vi "Main.vi"() -> ()   [LabVIEW 2020]
uses:
  Code/typeDefs/Parameters.ctl
  Code/typeDefs/MFCIn.ctl
  Code/typeDefs/MFCOut.ctl
  Code/typeDefs/keithleySettings.ctl
  Code/typeDefs/MFCSet.ctl
  <vilib>/Utility/miscctls.llb/LVPointTypeDef.ctl
  <vilib>/DAQmx/read.llb/DAQmx Read (Analog 2D DBL NChan NSamp).vi
  <vilib>/Analysis/baseanly.llb/Mean (DBL).vi
  <vilib>/DAQmx/write.llb/DAQmx Write (Digital 1D Bool NChan 1Samp 1Line).vi
  <vilib>/DAQmx/write.llb/DAQmx Write (Analog DBL 1Chan 1Samp).vi
  <vilib>/DAQmx/create/channels.llb/DAQmx Create Channel (AO-Voltage-Basic).vi
  <vilib>/DAQmx/miscellaneous.llb/DAQmx Fill In Error Info.vi
  <vilib>/DAQmx/create/channels.llb/DAQmx Create Channel (DO-Digital Output).vi
  <vilib>/DAQmx/create/channels.llb/DAQmx Create Channel (AI-Voltage-Basic).vi
  <vilib>/DAQmx/configure/timing.llb/DAQmx Timing (Sample Clock).vi
  <vilib>/Instr/_visa.llb/VISA Configure Serial Port (Instr).vi
  <vilib>/Analysis/NI_AALBase.lvlib
  <resource>/objmgr/daqmx.rc
  Code/DAQ/DAQ.lvclass
  Code/MFC/MFC.lvclass
  Code/SMU/SMU.lvclass
panel:
  out "Residue":dbl
  out "Intercept":dbl
  out "CvsV":T1(graph) caption="Current vs Voltage"
  in  "Timeout Stop":bool
  out "MFC Index":i32
  in  "Names":string[](array[string])=["Resistance (Ohms)", "Ethanol (%)", "RH (%)", "Temp (C)", "MFC A", "MFC B"]
  in  "Stop":bool
  in  "Tab Control":enum32{"Config", "Experiment", "Errors"}(tab)=enum."Experiment"
  in  "AO_LED":tag="6343Sim/ao0"
  in  "DO_Valves":tag="6343Sim/port0/line0:1"
  in  "DAQ channels":tag="6343Sim/ai0:2"
  in  "Keithley 2400 Name":refnum<visa-resource-name>
  in  "MFC Config":T2={"Tare absP"=FALSE, "Tare Flow"=FALSE, "Device ID's"=["A", "B"], "baud rate (9600)"=19200, "VISA COM Port"="COM3"}
  in  "DAQ Config":T3={"RH/T Sensor VSS (V)"=5.048, "K0"=0.9054, "K1"=-2.995, "Offset"=0.0, "Gain"=1.0, "Samples/Channel/s"=1000.0, "Samples to Average"=1000.0} {"Offset" step=0.01 format="%_3f"; "K1" format="%#_13g"; "K0" format="%#_13g"; "RH/T Sensor VSS (V)" format="%.3g"}
  out "Unprocessed Samples in Queue":u32=5
  out "DPS":dbl=100.0 caption="Data Points / Second"
  in  "Keithley Config":T4={"Source Compliance"=0.1, "Min Voltage"=0.0, "Max Voltage"=5.0, "Source Mode"=0, "Number of Points"=50} {"Source Mode" items=["Voltage", "Current"]}
  in  "Keithley Hz":u32=1 min=1 max=100 step=1
  in  "Hours to Run":dbl=1.0 min=0.25 max=10.0 step=0.25 format="%#_5g"
  in  "Aquire data":bool
  out "Start Time":timestamp format="%<%I:%M:%S %p>T"
  in  "MFC Set":T5[](array[typedef])=[{"MFC Set"=[{"String"="A", "MFC set"=1000.0}, {"String"="B", "MFC set"=100.0}], "set 1"=FALSE}, {"MFC Set"=[{"String"="A", "MFC set"=1000.0}, {"String"="B", "MFC set"=100.0}], "set 1"=TRUE}] {"MFC Set"."MFC set" step=10.0 format="%.2f"}
  in  "LED Voltage":dbl(slide) min=0.0 max=10.0 step=0.1 scale=0.0..10.0
  in  "Valves":bool[](array[boolean])=[FALSE, FALSE]
  in  "Plot Data":bool
  out "End Time":timestamp format="%<%I:%M:%S %p>T"
  in  "File Name":string
  in  "Save to File":bool
  out "LED_AO Error":errorcluster
  out "3-Valve_DO Error":errorcluster
  out "DAQ_IO Error":errorcluster
  out "MFC_IO Error":errorcluster
  out "Keithley Error":errorcluster
  in  "Clear I/V":bool
  out "Resistance (ohm)":dbl[](array[numeric])
  in  "Clear DAQ":bool
  out "Array":T6[](array[typedef])=[{"Gas"="", "Setpoint"=0.0, "MassFlow"=0.0, "T ºC"=0.0, "P(PSI)"=0.0, "ID"="-"}, {"Gas"="", "Setpoint"=0.0, "MassFlow"=0.0, "T ºC"=0.0, "P(PSI)"=0.0, "ID"="-"}] {"MassFlow" format="%.2f"; "Setpoint" format="%.2f"}
  out "Waveform Chart":waveform(dbl)[](graph)=[{"t0"=timestamp(3675342615.977705 s since 1904-01-01), "dt"=0.01, "Y"=[0.0007680409200236937]}, {"t0"=timestamp(3675342615.977705 s since 1904-01-01), "dt"=0.01, "Y"=[0.0105205510693704]}, {"t0"=timestamp(3675342615.977705 s since 1904-01-01), "dt"=0.01, "Y"=[89.00820200660893]}, {"t0"=timestamp(3675342615.977705 s since 1904-01-01), "dt"=0.01, "Y"=[117.62674839380017]}, {"t0"=timestamp(3675342615.977705 s since 1904-01-01), "dt"=0.01, "Y"=[0.0]}, {"t0"=timestamp(3675342615.977705 s since 1904-01-01), "dt"=0.01, "Y"=[0.0]}]
  out "T":dbl caption="T  (ºC)" format="%.2g"
  out "RH":dbl caption="RH  (%)" format="%.2g"
  out "Eth":dbl caption="Ethanol (%)" format="%.3g"
  # "Port Config"
  # "Save to File"
  # "1"
  # "2"
  # "1"
  # "2"
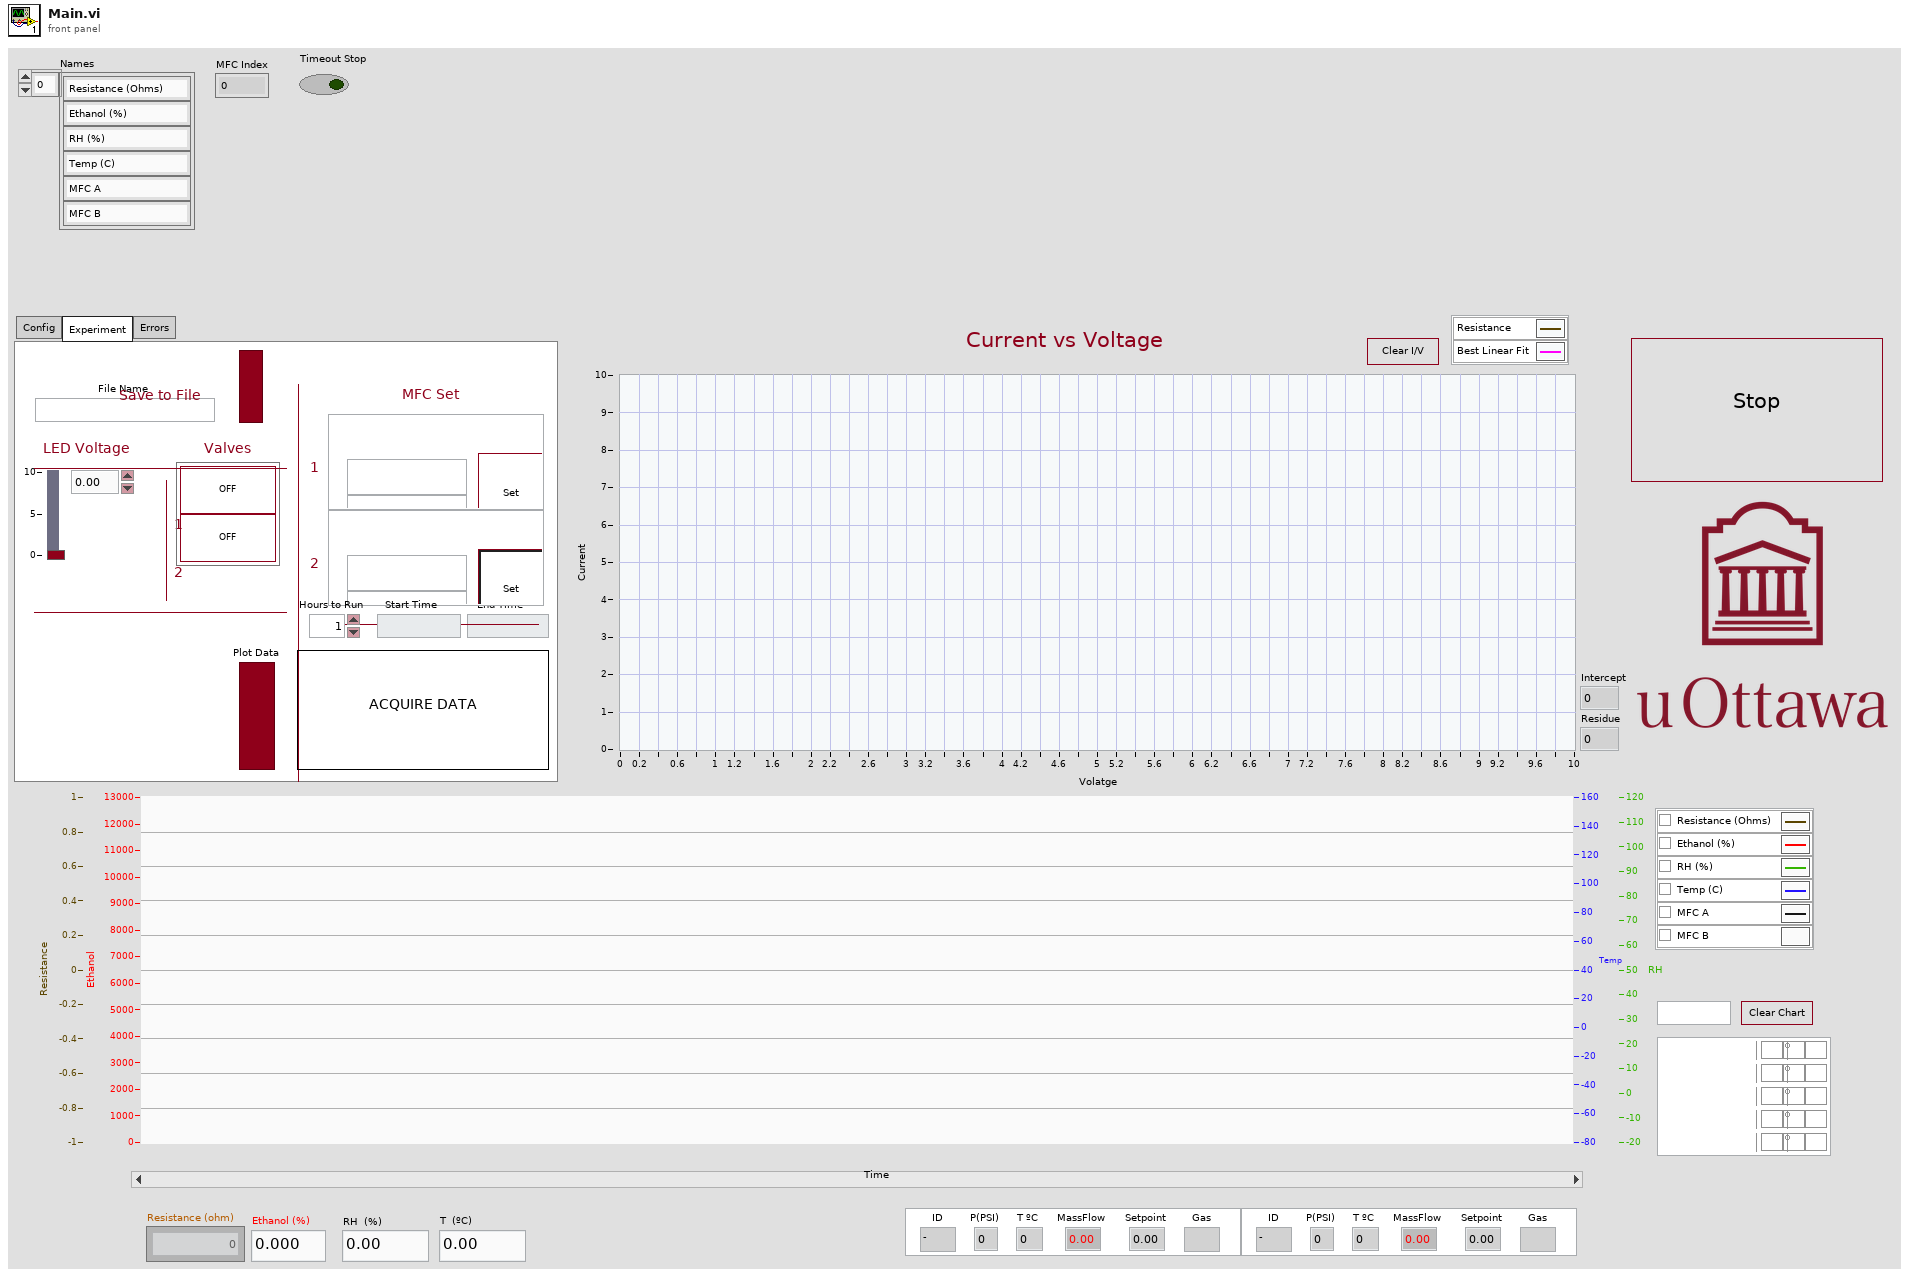
[diagram p1: front panel]
types:
  T1 = cluster{"array":sgl[], "Best Linear Fit":dbl[]}[]
  T2 = typedef "MFCIn.ctl" = cluster{"Tare absP":bool, "Tare Flow":bool, "Device ID's":string[], "baud rate (9600)":u32, "VISA COM Port":refnum<visa-resource-name>}
  T3 = typedef "Parameters.ctl" = cluster{"RH/T Sensor VSS (V)":dbl, "K0":dbl, "K1":dbl, "Offset":dbl, "Gain":dbl, "Samples/Channel/s":dbl, "Samples to Average":dbl}
  T4 = typedef "keithleySettings.ctl" = cluster{"Source Compliance":dbl, "Min Voltage":dbl, "Max Voltage":dbl, "Source Mode":u16, "Number of Points":u32}
  T5 = typedef "MFCSet.ctl" = cluster{"MFC Set":cluster{"String":string, "MFC set":dbl}[], "set 1":bool}
  T6 = typedef "MFCOut.ctl" = cluster{"Gas":string, "Setpoint":dbl, "MassFlow":dbl, "T ºC":dbl, "P(PSI)":dbl, "ID":string}
  T7 = typedef "LVPointTypeDef.ctl" = cluster{"Horizontal":i16, "Vertical":i16}
  T8 = enum8{"Enabled", "Disabled", "Disabled and Grayed Out"}
  T9 = enum32{"invalid app kind", "Development System", "Run Time System", "Student Edition", "Embedded LabVIEW", "Evaluation", "Custom"}
  T10 = cluster{"MFC Set":cluster{"String":bool, "MFC set":bool}[], "set 1":bool}
  T11 = typedef "Graph.ctl" = cluster{"Resistance":dbl, "Ethanol":dbl, "RH":dbl, "Temp":dbl, "MFC A":dbl, "MFC B":dbl}
  T12 = cluster{"ID":string, "P(PSI)":dbl, "T ºC":dbl, "MassFlow":dbl, "Setpoint":dbl, "Gas":string}[]
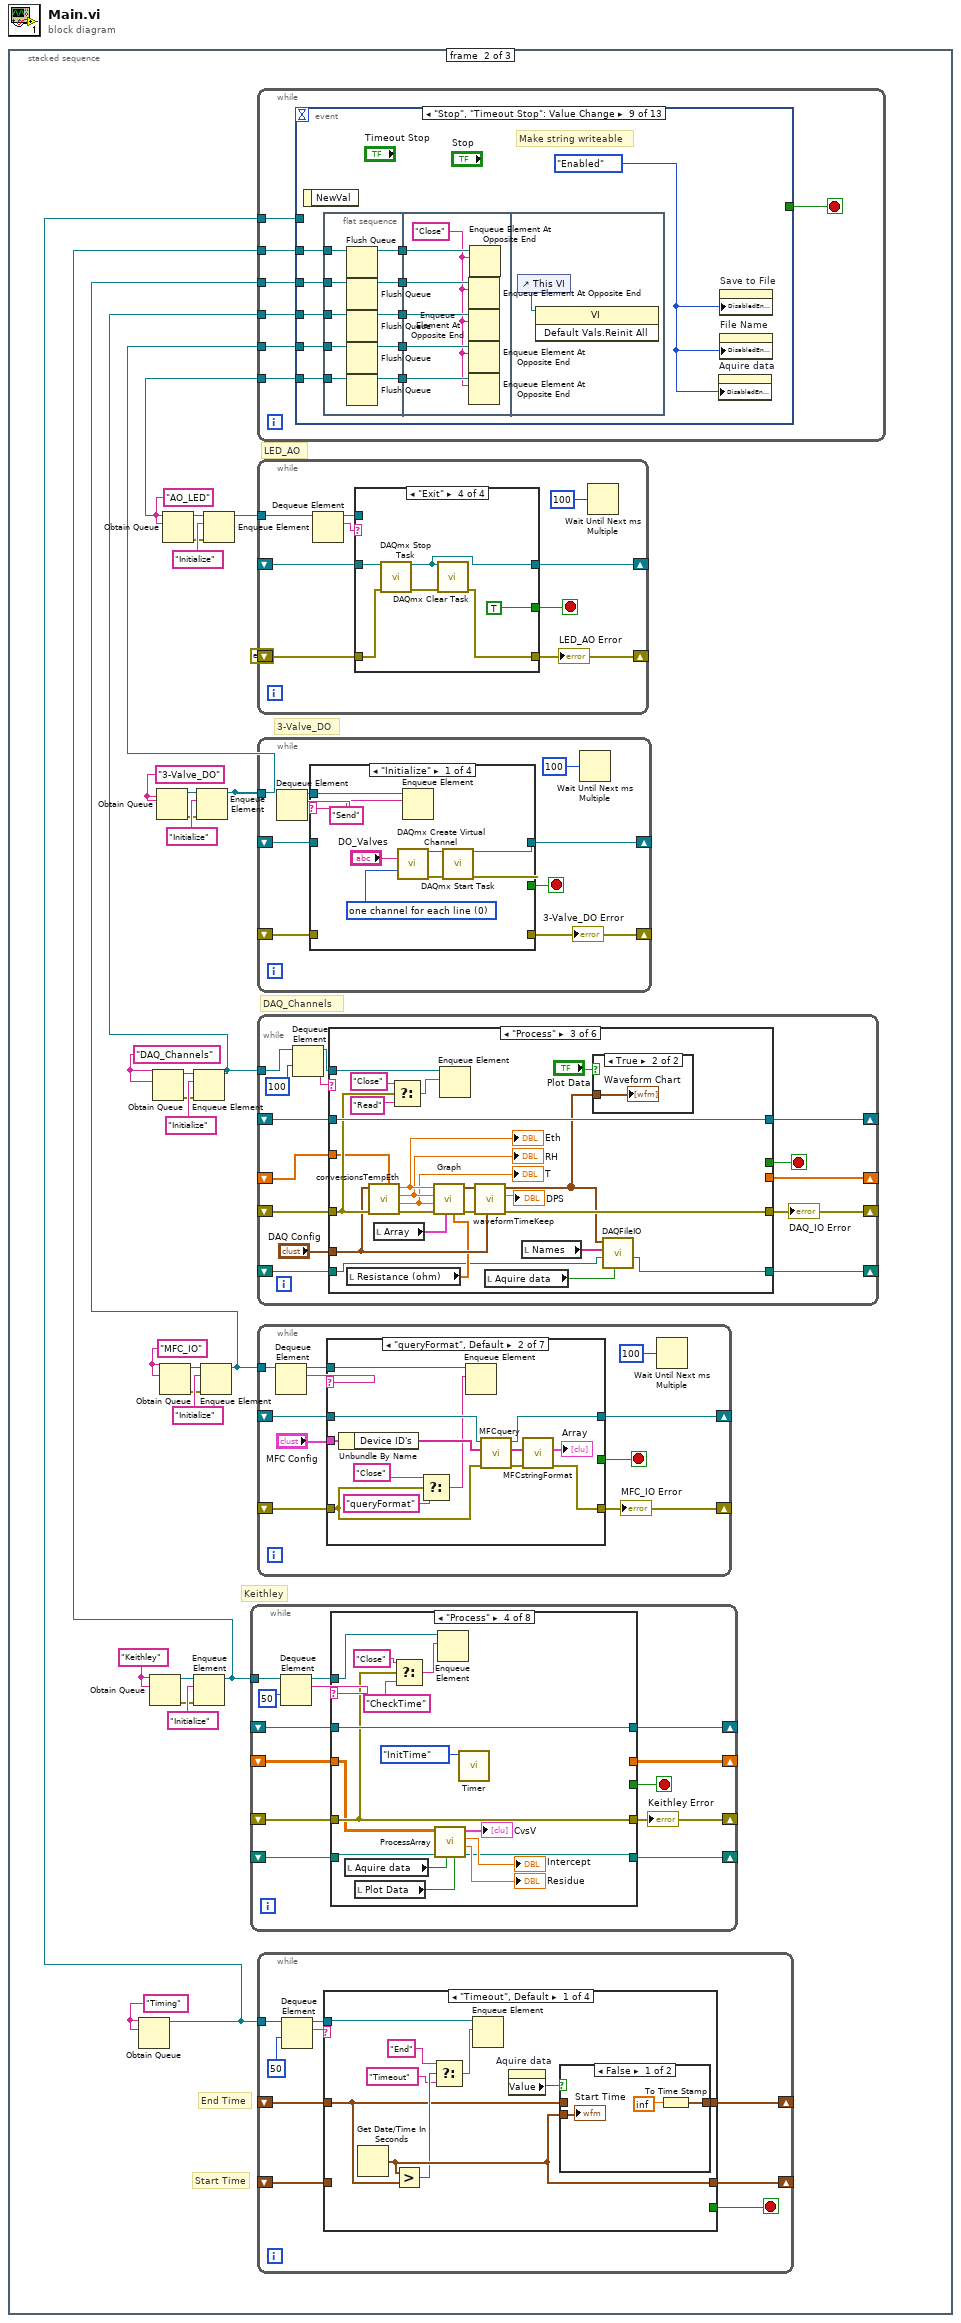
[diagram p0: block diagram]
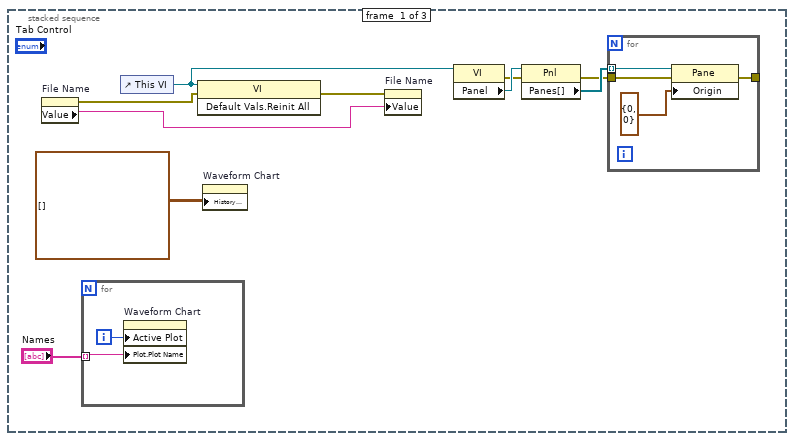
[diagram p2: hidden frame]
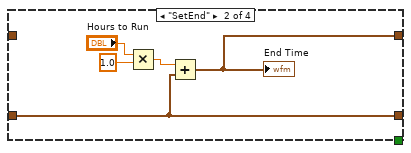
[diagram p4: hidden frame]
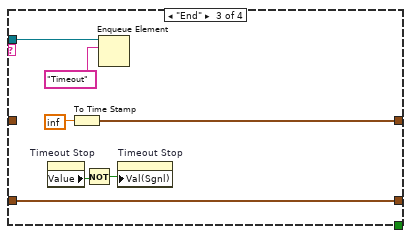
[diagram p5: hidden frame]
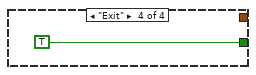
[diagram p6: hidden frame]
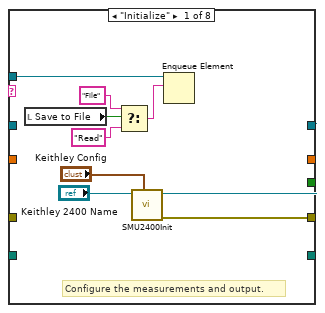
[diagram p7: hidden frame]
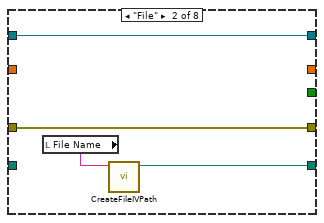
[diagram p8: hidden frame]
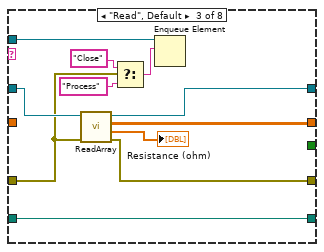
[diagram p9: hidden frame]
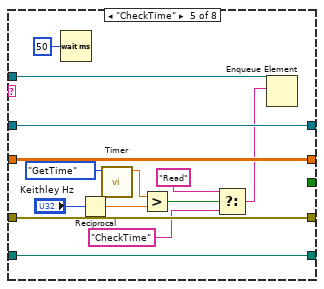
[diagram p10: hidden frame]
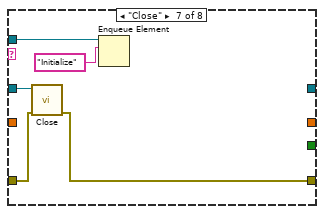
[diagram p12: hidden frame]
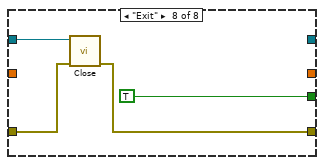
[diagram p13: hidden frame]
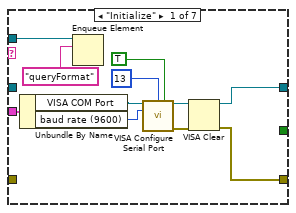
[diagram p14: hidden frame]
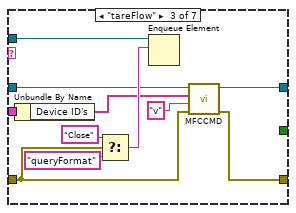
[diagram p15: hidden frame]
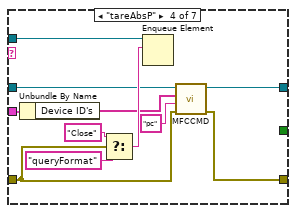
[diagram p16: hidden frame]
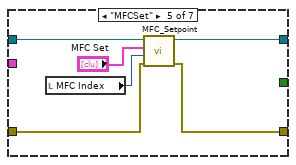
[diagram p17: hidden frame]
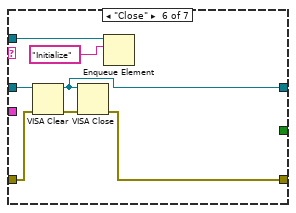
[diagram p18: hidden frame]
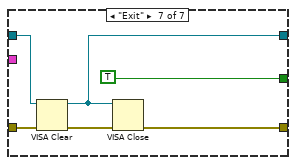
[diagram p19: hidden frame]
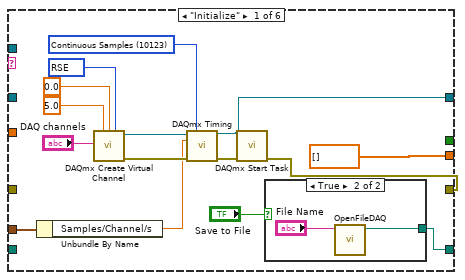
[diagram p20: hidden frame]
diagram:
  n1 = stacked-sequence {
    frame #0 {
      n2 = property on="File Name" class="Str"() -> (error out=w9:errorcluster, "Value"=w8:string)  [unwired: 2 in, 1 out]
      n3 = for {
        tunnel: "Names" -> [w15] mode=indexing
        i -> [w16]
        n4 = property on="Waveform Chart" class="WFChart (strict)"("Active Plot"=w16, "Plot.Plot Name"=w15) -> ()  [unwired: 2 in, 2 out]
      }
      n5 = control-ref of="This VI"() -> (w1:refnum<vi>)
      n6 = invoke class="VI" method="Default Vals.Reinit All"(reference=w1, error in=w9) -> (error out=w7:errorcluster)  [unwired: 1 in, 2 out]
      n7 = property on="Waveform Chart" class="WFChart (strict)"("History Data"=waveform(dbl)[][] []) -> ()  [unwired: 2 in, 2 out]
      n8 = property on="File Name" class="Str"(error in=w7, "Value"=w8) -> ()  [unwired: 1 in, 2 out]
      n9 = property class="VI"(reference=w1) -> (error out=w4:errorcluster, "Panel"=w5:refnum<vi>)  [unwired: 1 in, 1 out]
      n10 = property class="Pnl"(reference=w5, error in=w4) -> (error out=w2:errorcluster, "Panes[]"=w3:refnum<vi>[])  [unwired: 1 out]
      n11 = for {
        tunnel: w3 -> [w14] mode=indexing
        tunnel: w2 -> [w13]
        tunnel: [w11] -> _
        n12 = property class="Pane"(reference=w14, error in=w13, "Origin"=T7 {"Horizontal"=0, "Vertical"=0}) -> (error out=w11:errorcluster)  [unwired: 1 out]
      }
    }
    frame #1 {
      w18 = "Timing" ("name (unnamed)")
      w27 = "Keithley" ("name (unnamed)")
      w31 = "MFC_IO" ("name (unnamed)")
      w34 = "DAQ_Channels" ("name (unnamed)")
      w32 = "3-Valve_DO" ("name (unnamed)")
      w42 = "AO_LED" ("name (unnamed)")
      # "Start Time"
      # "End Time"
      # "Keithley"
      # "DAQ_Channels"
      # "3-Valve_DO"
      # "LED_AO"
      n13 = Obtain Queue(name (unnamed)=w18, element data type=w18) -> (queue out=w17:refnum<queue>)  [unwired: 3 in, 2 out]
      n14 = Obtain Queue(name (unnamed)=w27, element data type=w27) -> (queue out=w21:refnum<queue>, error out=w19:errorcluster)  [unwired: 3 in, 1 out]
      n15 = Obtain Queue(name (unnamed)=w34, element data type=w34) -> (queue out=w26:refnum<queue>, error out=w33:errorcluster)  [unwired: 3 in, 1 out]
      n16 = Obtain Queue(name (unnamed)=w32, element data type=w32) -> (queue out=w36:refnum<queue>, error out=w37:errorcluster)  [unwired: 3 in, 1 out]
      n17 = Obtain Queue(name (unnamed)=w31, element data type=w31) -> (queue out=w29:refnum<queue>, error out=w30:errorcluster)  [unwired: 3 in, 1 out]
      n18 = Obtain Queue(name (unnamed)=w42, element data type=w42) -> (queue out=w40:refnum<queue>, error out=w41:errorcluster)  [unwired: 3 in, 1 out]
      n19 = Enqueue Element(queue=w26, element="Initialize", error in (no error)=w33) -> (queue out=w25:refnum<queue>)  [unwired: 1 in, 2 out]
      n20 = Enqueue Element(queue=w21, element="Initialize", error in (no error)=w19) -> (queue out=w20:refnum<queue>)  [unwired: 1 in, 2 out]
      n21 = Enqueue Element(queue=w36, element="Initialize", error in (no error)=w37) -> (queue out=w22:refnum<queue>)  [unwired: 1 in, 2 out]
      n22 = Enqueue Element(queue=w29, element="Initialize", error in (no error)=w30) -> (queue out=w28:refnum<queue>)  [unwired: 1 in, 2 out]
      n23 = Enqueue Element(queue=w40, element="Initialize", error in (no error)=w41) -> (queue out=w23:refnum<queue>)  [unwired: 1 in, 2 out]
      n24 = while {
        shift-right: [w86] -> _
        shift-left: _ -> [w90]
        shift-right: [w89] -> _
        shift-left: _ -> [w88]
        tunnel: w20 -> [w87]
        shift-right: [w84] -> _
        shift-left: _ -> [w83]
        shift-right: [w82] -> _
        shift-left: _ -> [w81]
        stop <- w85 stop-if-true
        n25 = Dequeue Element(queue=w87, timeout in ms (-1)=50) -> (queue out=w92:refnum<queue>, element=w91:string)  [unwired: 1 in, 2 out]
        n26 = case shown="\"Process\"" w91 {
          tunnel: w92 -> [w101 _ w116 w129 w132 _ w152 _]
          tunnel: [_ _ _ _ _ _ _ TRUE] -> w85
          tunnel: [w94 w105 w107 w126 w145 w148 w151 w155] -> w86
          tunnel: w90 -> [_ w105 w106 w126 w145 w148 w150 w154]
          tunnel: [w93 w103 w109 w127 w138 w147 _ _] -> w89
          tunnel: w88 -> [_ w103 w110 w127 w138 w147 w149 w156]
          tunnel: [_ _ w111 _ w137 _ _ _] -> w84
          tunnel: w83 -> [_ _ _ w123 w137 _ _ _]
          tunnel: [_ w102 w112 w117 w139 w146 _ _] -> w82
          tunnel: w81 -> [_ _ w112 w124 w139 w146 _ _]
          frame "Initialize" {
            # "Configure the measurements and output."
            n27 = local read "Save to File"() -> (w98:bool)
            n28 = Select(t="File", s=w98, f="Read" ("element")) -> (s? t:f=w97:string)
            n29 = call "SMU2400Init.vi"("Keithley Config"="Keithley Config", "Keithley 2400 Name"="Keithley 2400 Name") -> ("error out"=w94:errorcluster, "VISA resource name out"=w93:refnum<visa-resource-name>)  [unwired: 8 in]
            n30 = Enqueue Element(queue=w101, element=w97) -> ()  [unwired: 2 in, 3 out]
          }
          frame "File" {
            n31 = local read "File Name"() -> (w104:string)
            n32 = call "CreateFileIVPath.vi"("File Name"=w104) -> ("appended path"=w102:path)  [unwired: 9 in, 1 out]
          }
          frame "Read", Default {
            n33 = call "ReadArray.vi"("error in (no error)"=w106, "VISA resource name"=w110) -> ("error out"=w107:errorcluster, "Resistance (ohm)"=→"Resistance (ohm)":dbl[], "appended array"=w111:sgl[][], "VISA resource name out"=w109:refnum<visa-resource-name>)  [unwired: 6 in]
            n34 = Select(t="Close" ("element"), s=w106, f="Process" ("element")) -> (s? t:f=w114:string)
            n35 = Enqueue Element(queue=w116, element=w114) -> ()  [unwired: 2 in, 3 out]
          }
          frame "Process" {
            n36 = local read "Aquire data"() -> (w121:bool)
            n37 = local read "Plot Data"() -> (w120:bool)
            n38 = Select(t="Close" ("element"), s=w126, f="CheckTime" ("element")) -> (s? t:f=w128:string)
            n39 = call "ProcessArray.vi"("Plot Data"=w120, "Aquire Data"=w121, "File Path In"=w124, "array in"=w123) -> ("file path out"=w117:path, "residue"=→"Residue":dbl, "intercept"=→"Intercept":dbl, "Array out"=→"CvsV":T1)  [unwired: 4 in]
            n40 = Enqueue Element(queue=w129, element=w128) -> ()  [unwired: 2 in, 3 out]
            n41 = call "Timer.vi"("State"=enum16{"GetTime", "InitTime"}."InitTime") -> ()  [unwired: 10 in, 1 out]
          }
          frame "CheckTime" {
            n42 = Wait (ms)(milliseconds to wait=u32 50) -> ()  [unwired: 1 out]
            n43 = Reciprocal(x="Keithley Hz") -> (1/x=w141:dbl)
            n44 = call "Timer.vi"("State"=enum16{"GetTime", "InitTime"}."GetTime") -> ("Timer (s)"=w142:dbl)  [unwired: 10 in]
            n45 = Greater?(x=w142, y=w141) -> (0:w136:bool)
            n46 = Select(t="Read", s=w136, f="CheckTime") -> (s? t:f=w133:string)
            n47 = Enqueue Element(queue=w132, element=w133) -> ()  [unwired: 2 in, 3 out]
          }
          frame "Clear" {
          }
          frame "Close" {
            n48 = call "Close.vi"("error in (no error)"=w150, "VISA resource name"=w149) -> ("error out"=w151:errorcluster)  [unwired: 8 in, 1 out]
            n49 = Enqueue Element(queue=w152, element="Initialize") -> ()  [unwired: 2 in, 3 out]
          }
          frame "Exit" {
            n50 = call "Close.vi"("error in (no error)"=w154, "VISA resource name"=w156) -> ("error out"=w155:errorcluster)  [unwired: 8 in, 1 out]
          }
        }
        "Keithley Error" <- w86
      }
      n51 = while {
        tunnel: w23 -> [w408]
        tunnel: w22 -> [w407]
        tunnel: w25 -> [w406]
        tunnel: w28 -> [w405]
        tunnel: w20 -> [w404]
        tunnel: w17 -> [w403]
        stop <- w409 stop-if-true
        n52 = event shown="[8] \"Stop\", \"Timeout Stop\": Value Change" {
          selector: _ -> [_ _ _ _ _ _ _ _ _ _ _ _ _]
          dyn-events: _ -> [_ _ _ _ _ _ _ _ _ _ _ _ _]
          timeout: _ -> [_ _ _ _ _ _ _ _ _ _ _ _ _]
          tunnel: [_ _ w416 _ _ _ _ _ _ _ _ _ _] -> w409
          tunnel: w408 -> [_ _ w417 _ _ _ _ _ w457 _ _ _ _]
          tunnel: w407 -> [_ _ w418 _ _ _ _ _ w458 _ _ _ _]
          tunnel: w406 -> [_ _ w419 w433 w437 _ _ _ w459 _ w492 w503 w517]
          tunnel: w405 -> [_ _ w420 _ _ _ w448 w449 w460 w480 _ _ _]
          tunnel: w404 -> [_ _ w421 _ w435 w446 _ _ w461 _ w491 w502 w518]
          tunnel: w403 -> [_ w410 w415 _ _ _ _ _ _ _ _ _ _]
          event Timeout {
            n53 = event-data() -> ()  [unwired: 1 in, 1 out]
          }
          event "Aquire data": Value Change {
            n54 = event-data() -> ("NewVal"=w411:bool)  [unwired: 1 in]
            n55 = case shown="True" w411 {
              tunnel: w410 -> [_ w413]
              frame False {
              }
              frame True {
                w412 = T8."Disabled and Grayed Out" ("Disabled")
                n56 = Enqueue Element(queue=w413, element="SetEnd") -> ()  [unwired: 2 in, 3 out]
                n57 = property on="File Name" class="Str"("DisabledEnum"=w412) -> ()  [unwired: 2 in, 2 out]
                n58 = property on="Aquire data" class="Bool (strict)"("DisabledEnum"=w412) -> ()  [unwired: 2 in, 2 out]
                n59 = property on="Save to File" class="Bool (strict)"("DisabledEnum"=w412) -> ()  [unwired: 2 in, 2 out]
              }
            }
          }
          event Panel Close? {
            n60 = event-data() -> ()  [unwired: 1 in, 1 out]
            n61 = Two Button Dialog(message="Are you sure you would like to close?", 2:"Yes" ("T button name (\"OK\")")) -> (T button?=w416:bool)  [unwired: 1 in]
            n62 = case shown="True" w416 {
              tunnel: w421 -> [_ w431]
              tunnel: w420 -> [_ w430]
              tunnel: w419 -> [_ w429]
              tunnel: w418 -> [_ w428]
              tunnel: w417 -> [_ w427]
              tunnel: w415 -> [_ w426]
              frame False {
              }
              frame True {
                w425 = "Exit" ("element")
                n63 = Enqueue Element At Opposite End(queue=w430, element=w425) -> ()  [unwired: 2 in, 3 out]
                n64 = Enqueue Element At Opposite End(queue=w429, element=w425) -> ()  [unwired: 2 in, 3 out]
                n65 = Enqueue Element At Opposite End(queue=w428, element=w425) -> ()  [unwired: 2 in, 3 out]
                n66 = Enqueue Element At Opposite End(queue=w427, element=w425) -> ()  [unwired: 2 in, 3 out]
                n67 = Enqueue Element At Opposite End(queue=w426, element=w425) -> ()  [unwired: 2 in, 3 out]
                n68 = Enqueue Element At Opposite End(queue=w431, element=w425) -> ()  [unwired: 2 in, 3 out]
              }
            }
            n69 = event-data("Discard?"=TRUE) -> ()  [unwired: 1 in, 1 out]
          }
          event "Clear DAQ": Value Change {
            n70 = event-data() -> ()  [unwired: 1 in, 1 out]
            n71 = Enqueue Element(queue=w433, element="Clear") -> ()  [unwired: 2 in, 3 out]
          }
          event Value Change {
            n72 = event-data() -> ()  [unwired: 1 in, 1 out]
            n73 = flat-sequence {
              tunnel: w437 -> [w441]
              tunnel: [w440] -> w436
              tunnel: w435 -> [w439]
              tunnel: [w438] -> w434
              tunnel: w436 -> [w444]
              tunnel: w434 -> [w443]
              frame #0 {
                n74 = Flush Queue(queue=w441) -> (queue out=w440:refnum<queue>)  [unwired: 1 in, 2 out]
                n75 = Flush Queue(queue=w439) -> (queue out=w438:refnum<queue>)  [unwired: 1 in, 2 out]
              }
              frame #1 {
                w442 = "Close" ("element")
                n76 = Enqueue Element(queue=w444, element=w442) -> ()  [unwired: 2 in, 3 out]
                n77 = Enqueue Element(queue=w443, element=w442) -> ()  [unwired: 2 in, 3 out]
              }
            }
          }
          event "Clear I/V": Value Change {
            n78 = event-data() -> ()  [unwired: 1 in, 1 out]
            n79 = Enqueue Element(queue=w446, element="Clear") -> ()  [unwired: 2 in, 3 out]
          }
          event Value Change {
            n80 = event-data() -> ()  [unwired: 1 in, 6 out]
            n81 = Enqueue Element(queue=w448, element="tareFlow") -> ()  [unwired: 2 in, 3 out]
          }
          event Value Change {
            n82 = event-data() -> ()  [unwired: 1 in, 1 out]
            n83 = Enqueue Element(queue=w449, element="tareAbsP") -> ()  [unwired: 2 in, 3 out]
          }
          event "Stop", "Timeout Stop": Value Change {
            w451 = T8."Enabled" ("Disabled")
            # "Make string writeable"
            n84 = event-data() -> ()  [unwired: 1 in, 1 out]
            n85 = flat-sequence {
              tunnel: w457 -> [w463]
              tunnel: w458 -> [w465]
              tunnel: w459 -> [w467]
              tunnel: w460 -> [w469]
              tunnel: w461 -> [w471]
              tunnel: [w470] -> w456
              tunnel: [w468] -> w455
              tunnel: [w466] -> w454
              tunnel: [w464] -> w453
              tunnel: [w462] -> w452
              tunnel: w456 -> [w477]
              tunnel: w455 -> [w473]
              tunnel: w454 -> [w474]
              tunnel: w453 -> [w475]
              tunnel: w452 -> [w476]
              frame #0 {
                n86 = Flush Queue(queue=w471) -> (queue out=w470:refnum<queue>)  [unwired: 1 in, 2 out]
                n87 = Flush Queue(queue=w469) -> (queue out=w468:refnum<queue>)  [unwired: 1 in, 2 out]
                n88 = Flush Queue(queue=w467) -> (queue out=w466:refnum<queue>)  [unwired: 1 in, 2 out]
                n89 = Flush Queue(queue=w465) -> (queue out=w464:refnum<queue>)  [unwired: 1 in, 2 out]
                n90 = Flush Queue(queue=w463) -> (queue out=w462:refnum<queue>)  [unwired: 1 in, 2 out]
              }
              frame #1 {
                w472 = "Close" ("element")
                n91 = Enqueue Element At Opposite End(queue=w473, element=w472) -> ()  [unwired: 2 in, 3 out]
                n92 = Enqueue Element At Opposite End(queue=w474, element=w472) -> ()  [unwired: 2 in, 3 out]
                n93 = Enqueue Element At Opposite End(queue=w475, element=w472) -> ()  [unwired: 2 in, 3 out]
                n94 = Enqueue Element At Opposite End(queue=w476, element=w472) -> ()  [unwired: 2 in, 3 out]
                n95 = Enqueue Element At Opposite End(queue=w477, element=w472) -> ()  [unwired: 2 in, 3 out]
              }
              frame #2 {
                n96 = control-ref of="This VI"() -> (w478:refnum<vi>)
                n97 = invoke class="VI" method="Default Vals.Reinit All"(reference=w478) -> ()  [unwired: 2 in, 3 out]
              }
            }
            n98 = property on="Aquire data" class="Bool (strict)"("DisabledEnum"=w451) -> ()  [unwired: 2 in, 2 out]
            n99 = property on="Save to File" class="Bool (strict)"("DisabledEnum"=w451) -> ()  [unwired: 2 in, 2 out]
            n100 = property on="File Name" class="Str"("DisabledEnum"=w451) -> ()  [unwired: 2 in, 2 out]
          }
          event "MFC Set": Value Change {
            n101 = event-data() -> ("OldVal"=w481:T5[], "NewVal"=w479:T5[])  [unwired: 1 in]
            n102 = for {
              tunnel: w481 -> [w487] mode=indexing
              tunnel: w480 -> [w483]
              tunnel: w479 -> [w482] mode=indexing
              i -> [w485]
              stop <- w484 stop-if-true
              n103 = Not Equal?(x=w487, y=w482) -> (x != y?=w486:T10)
              n104 = Unbundle(w486) -> ("set 1"=w484:bool)  [unwired: 1 out]
              n105 = case shown="True" w484 {
                tunnel: w483 -> [_ w488]
                frame False {
                }
                frame True {
                  n106 = Enqueue Element(queue=w488, element="MFCSet") -> ()  [unwired: 2 in, 3 out]
                }
              }
              "MFC Index" <- w485
            }
          }
          event "File Name": Value Change {
            n107 = event-data() -> ()  [unwired: 1 in, 1 out]
            n108 = flat-sequence {
              tunnel: w492 -> [w497]
              tunnel: [w496] -> w493
              tunnel: w491 -> [w495]
              tunnel: [w494] -> w490
              tunnel: w493 -> [w500]
              tunnel: w490 -> [w499]
              frame #0 {
                n109 = Flush Queue(queue=w497) -> (queue out=w496:refnum<queue>)  [unwired: 1 in, 2 out]
                n110 = Flush Queue(queue=w495) -> (queue out=w494:refnum<queue>)  [unwired: 1 in, 2 out]
              }
              frame #1 {
                w498 = "Close" ("element")
                n111 = Enqueue Element(queue=w500, element=w498) -> ()  [unwired: 2 in, 3 out]
                n112 = Enqueue Element(queue=w499, element=w498) -> ()  [unwired: 2 in, 3 out]
              }
            }
          }
          event "Save to File": Value Change {
            n113 = event-data() -> ("NewVal"=w506:bool)  [unwired: 1 in]
            n114 = flat-sequence {
              tunnel: w503 -> [w510]
              tunnel: [w509] -> w504
              tunnel: w502 -> [w508]
              tunnel: [w507] -> w501
              tunnel: w504 -> [w513]
              tunnel: w501 -> [w512]
              frame #0 {
                n115 = Flush Queue(queue=w510) -> (queue out=w509:refnum<queue>)  [unwired: 1 in, 2 out]
                n116 = Flush Queue(queue=w508) -> (queue out=w507:refnum<queue>)  [unwired: 1 in, 2 out]
              }
              frame #1 {
                w511 = "Close" ("element")
                n117 = Enqueue Element(queue=w512, element=w511) -> ()  [unwired: 2 in, 3 out]
                n118 = Enqueue Element(queue=w513, element=w511) -> ()  [unwired: 2 in, 3 out]
              }
            }
            n119 = case shown="False" w506 {
              tunnel: [T8."Enabled" ("Disabled") T8."Disabled and Grayed Out" ("Disabled")] -> w505
              frame False {
              }
              frame True {
              }
            }
            n120 = property on="File Name" class="Str"("DisabledEnum"=w505) -> ()  [unwired: 2 in, 2 out]
          }
          event Value Change {
            n121 = event-data() -> ()  [unwired: 1 in, 1 out]
            n122 = flat-sequence {
              tunnel: w518 -> [w523]
              tunnel: [w522] -> w519
              tunnel: w517 -> [w521]
              tunnel: [w520] -> w516
              tunnel: w519 -> [w526]
              tunnel: w516 -> [w525]
              frame #0 {
                n123 = Flush Queue(queue=w523) -> (queue out=w522:refnum<queue>)  [unwired: 1 in, 2 out]
                n124 = Flush Queue(queue=w521) -> (queue out=w520:refnum<queue>)  [unwired: 1 in, 2 out]
              }
              frame #1 {
                w524 = "Close" ("element")
                n125 = Enqueue Element(queue=w525, element=w524) -> ()  [unwired: 2 in, 3 out]
                n126 = Enqueue Element(queue=w526, element=w524) -> ()  [unwired: 2 in, 3 out]
              }
            }
          }
        }
      }
      n127 = while {
        shift-right: [w367] -> _
        shift-left: errorcluster {"status"=FALSE, "code"=0, "source"=""} ("error out") -> [w370]
        shift-right: [w369] -> _
        shift-left: _ -> [w368]
        tunnel: w23 -> [w366]
        stop <- w371 stop-if-true
        n128 = Dequeue Element(queue=w366) -> (queue out=w373:refnum<queue>, element=w372:string)  [unwired: 2 in, 2 out]
        n129 = case shown="\"Exit\"" w372 {
          tunnel: w373 -> [w380 w389 w395 _]
          tunnel: [_ _ _ TRUE] -> w371
          tunnel: [w377 w386 w392 w400] -> w367
          tunnel: w370 -> [_ w385 w390 w398]
          tunnel: [w378 w387 w393 w397] -> w369
          tunnel: w368 -> [_ w388 w394 w401]
          frame "Initialize" {
            n130 = Enqueue Element(queue=w380, element="Send") -> ()  [unwired: 2 in, 3 out]
            n131 = call-poly <vilib>:"DAQmx Create Virtual Channel.vi"("physical channels"="AO_LED") -> ("task out"=w376:refnum<k21>, "error out"=w375:errorcluster)  [unwired: 13 in]
            n132 = call <vilib>:"DAQmx Start Task.vi"("task/channels in"=w376, "error in"=w375) -> ("task out"=w378:refnum<k21>, "error out"=w377:errorcluster)  [unwired: 12 in]
          }
          frame "Send", Default {
            n133 = Select(t="Close" ("element"), s=w385, f="Send" ("element")) -> (s? t:f=w382:string)
            n134 = call-poly <vilib>:"DAQmx Write.vi"("task/channels in"=w388, "data"="LED Voltage", "error in"=w385) -> ("task out"=w387:refnum<k21>, "error out"=w386:errorcluster)  [unwired: 10 in, 1 out]
            n135 = Enqueue Element(queue=w389, element=w382) -> ()  [unwired: 2 in, 3 out]
          }
          frame "Close" {
            n136 = call <vilib>:"DAQmx Stop Task.vi"("task/channels in"=w394, "error in"=w390) -> ("task out"=w393:refnum<k21>, "error out"=w391:errorcluster)  [unwired: 12 in]
            n137 = call <vilib>:"DAQmx Clear Task.vi"("task in"=w393, "error in"=w391) -> ("error out"=w392:errorcluster)  [unwired: 13 in]
            n138 = Enqueue Element(queue=w395, element="Initialize") -> ()  [unwired: 2 in, 3 out]
          }
          frame "Exit" {
            n139 = call <vilib>:"DAQmx Stop Task.vi"("task/channels in"=w401, "error in"=w398) -> ("task out"=w397:refnum<k21>, "error out"=w399:errorcluster)  [unwired: 12 in]
            n140 = call <vilib>:"DAQmx Clear Task.vi"("task in"=w397, "error in"=w399) -> ("error out"=w400:errorcluster)  [unwired: 13 in]
          }
        }
        "LED_AO Error" <- w367
        n141 = Wait Until Next ms Multiple(millisecond multiple=u32 100) -> ()  [unwired: 1 out]
      }
      n142 = while {
        shift-right: [w327] -> _
        shift-left: _ -> [w330]
        shift-right: [w329] -> _
        shift-left: _ -> [w328]
        tunnel: w22 -> [w326]
        stop <- w332 stop-if-true
        n143 = Dequeue Element(queue=w326) -> (queue out=w334:refnum<queue>, element=w333:string)  [unwired: 2 in, 2 out]
        n144 = case shown="\"Initialize\"" w333 {
          tunnel: w334 -> [w342 w351 w357 _]
          tunnel: [_ _ _ TRUE] -> w332
          tunnel: [w339 w348 w354 w361] -> w327
          tunnel: w330 -> [_ w347 w352 w359]
          tunnel: [w340 w349 w355 w362] -> w329
          tunnel: w328 -> [_ w350 w356 w363]
          frame "Initialize" {
            w336 = 0 items=["one channel for each line", "one channel for all lines"] ("line grouping")
            n145 = call-poly <vilib>:"DAQmx Create Virtual Channel.vi"("lines"="DO_Valves", "line grouping"=w336) -> ("task out"=w338:refnum<k21>, "error out"=w337:errorcluster)  [unwired: 12 in]
            n146 = Enqueue Element(queue=w342, element="Send") -> ()  [unwired: 2 in, 3 out]
            n147 = call <vilib>:"DAQmx Start Task.vi"("task/channels in"=w338, "error in"=w337) -> ("task out"=w340:refnum<k21>, "error out"=w339:errorcluster)  [unwired: 12 in]
          }
          frame "Send", Default {
            n148 = Select(t="Close" ("element"), s=w347, f="Send" ("element")) -> (s? t:f=w344:string)
            n149 = Enqueue Element(queue=w351, element=w344) -> ()  [unwired: 2 in, 3 out]
            n150 = call-poly <vilib>:"DAQmx Write.vi"("task/channels in"=w350, "data"="Valves", "error in"=w347) -> ("task out"=w349:refnum<k21>, "error out"=w348:errorcluster)  [unwired: 10 in, 1 out]
          }
          frame "Close" {
            n151 = call <vilib>:"DAQmx Stop Task.vi"("task/channels in"=w356, "error in"=w352) -> ("task out"=w355:refnum<k21>, "error out"=w353:errorcluster)  [unwired: 12 in]
            n152 = call <vilib>:"DAQmx Clear Task.vi"("task in"=w355, "error in"=w353) -> ("error out"=w354:errorcluster)  [unwired: 13 in]
            n153 = Enqueue Element(queue=w357, element="Initialize") -> ()  [unwired: 2 in, 3 out]
          }
          frame "Exit" {
            n154 = call <vilib>:"DAQmx Stop Task.vi"("task/channels in"=w363, "error in"=w359) -> ("task out"=w362:refnum<k21>, "error out"=w360:errorcluster)  [unwired: 12 in]
            n155 = call <vilib>:"DAQmx Clear Task.vi"("task in"=w362, "error in"=w360) -> ("error out"=w361:errorcluster)  [unwired: 13 in]
          }
        }
        "3-Valve_DO Error" <- w327
        n156 = Wait Until Next ms Multiple(millisecond multiple=u32 100) -> ()  [unwired: 1 out]
      }
      n157 = while {
        shift-right: [w241] -> _
        shift-left: _ -> [w244]
        shift-right: [w243] -> _
        shift-left: _ -> [w242]
        shift-right: [w240] -> _
        shift-left: _ -> [w238]
        tunnel: w25 -> [w239]
        shift-right: [w234] -> _
        shift-left: _ -> [w233]
        stop <- w236 stop-if-true
        n158 = Dequeue Element(queue=w239, timeout in ms (-1)=100) -> (queue out=w246:refnum<queue>, element=w245:string)  [unwired: 1 in, 2 out]
        n159 = case shown="\"Process\"" w245 {
          tunnel: w246 -> [_ w273 w304 _ w315 _]
          tunnel: [_ _ _ _ _ TRUE] -> w236
          tunnel: [w248 w267 w294 w311 w313 w323] -> w241
          tunnel: w244 -> [_ w270 w301 w309 w314 w320]
          tunnel: [w254 w276 w302 w312 _ _] -> w243
          tunnel: w242 -> [_ w278 w302 w312 w316 w324]
          tunnel: [dbl[] [] w269 _ dbl[] [] _ _] -> w240
          tunnel: w238 -> [_ _ w292 _ _ _]
          tunnel: "DAQ Config" -> [w252 w265 w289 _ _ _]
          tunnel: [w247 w264 w285 w307 _ _] -> w234
          tunnel: w233 -> [_ w264 w282 w307 _ _]
          frame "Initialize" {
            w257 = 10123 items=["Finite Samples"=10178, "Continuous Samples"=10123, "Hardware Timed Single Point"=12522] ("sample mode")
            w250 = 10083 items=["default"=-1, "RSE"=10083, "NRSE"=10078, "Differential"=10106, "Pseudodifferential"=12529] ("input terminal configuration")
            n160 = Unbundle By Name(w252) -> ("Samples/Channel/s"=w251:dbl)
            n161 = call-poly <vilib>:"DAQmx Create Virtual Channel.vi"("maximum value"=5.0, "minimum value"=0.0, "input terminal configuration"=w250, "physical channels"="DAQ channels") -> ("task out"=w258:refnum<k21>, "error out"=w259:errorcluster)  [unwired: 10 in]
            n162 = call-poly <vilib>:"DAQmx Timing.vi"("task/channels in"=w258, "sample mode"=w257, "rate"=w251, "error in"=w259) -> ("task out"=w254:refnum<k21>, "error out"=w260:errorcluster)  [unwired: 10 in]
            n163 = call <vilib>:"DAQmx Start Task.vi"("task/channels in"=w254, "error in"=w260) -> ("error out"=w248:errorcluster)  [unwired: 12 in, 1 out]
            n164 = case shown="True" "Save to File" {
              tunnel: [_ w262] -> w247
              frame False {
              }
              frame True {
                n165 = call "OpenFileDAQ.vi"("DAQ File Name"="File Name") -> ("appended path"=w262:path)  [unwired: 8 in, 1 out]
              }
            }
          }
          frame "Read", Default {
            n166 = Unbundle By Name(w265) -> ("Samples to Average"=w275:dbl)
            n167 = property class="DAQmx Read"(reference=w278, error in=w270) -> (reference out=w277:refnum<k21>, error out=w274:errorcluster, "AvailSampPerChan"=→"Unprocessed Samples in Queue":u32)
            n168 = Select(t="Close" ("element"), s=w270, f="Process" ("element")) -> (s? t:f=w279:string)
            n169 = Enqueue Element(queue=w273, element=w279) -> ()  [unwired: 2 in, 3 out]
            n170 = call-poly <vilib>:"DAQmx Read.vi"("task/channels in"=w277, "number of samples per channel"=w275, "error in"=w274) -> ("task out"=w276:refnum<k21>, "data"=w268:dbl[][], "error out"=w267:errorcluster)  [unwired: 10 in]
            n171 = for {
              tunnel: w268 -> [w280] mode=indexing
              tunnel: [w281] -> w269 mode=indexing
              n172 = call-poly <vilib>:"Mean.vi"("X"=w280) -> ("mean"=w281:dbl)  [unwired: 1 out]
            }
          }
          frame "Process" {
            n173 = local read "Resistance (ohm)"() -> (w287:dbl[])
            n174 = call "conversionsTempEth.vi"("Array"=w292, "error in (no error)"=w301, "Parameters"=w289) -> ("error out"=w299:errorcluster, "T"=w296:dbl, "RH"=w297:dbl, "Ethanol"=w298:dbl)  [unwired: 5 in]
            "Eth" <- w298
            "RH" <- w297
            "T" <- w296
            n175 = local read "Array"() -> (w300:T6[])
            n176 = Select(t="Close" ("element"), s=w301, f="Read") -> (s? t:f=w303:string)
            n177 = call "Graph.vi"("Resistance"=w287, "Array in"=w300, "error in (no error)"=w299, "T  (ºC)"=w296, "RH  (%)"=w297, "Ethanol (%)"=w298) -> ("error out"=w295:errorcluster, "Cluster"=w293:T11)  [unwired: 4 in]
            n178 = Enqueue Element(queue=w304, element=w303) -> ()  [unwired: 2 in, 3 out]
            n179 = call "waveformTimeKeep.vi"("DAQ Settings"=w289, "error in (no error)"=w295, "input cluster"=w293) -> ("error out"=w294:errorcluster, "Samples/second"=→"DPS":dbl, "appended array"=w283:waveform(dbl)[])  [unwired: 6 in]
            n180 = local read "Aquire data"() -> (w286:bool)
            n181 = local read "Names"() -> (w284:string[])
            n182 = case shown="True" "Plot Data" {
              tunnel: w283 -> [_ w306]
              frame False {
              }
              frame True {
                "Waveform Chart" <- w306
              }
            }
            n183 = call "DAQFileIO.vi"("Aquire Data"=w286, "File Path In"=w282, "Names"=w284, "data"=w283) -> ("file path out"=w285:path)  [unwired: 6 in, 1 out]
          }
          frame "Clear" {
            n184 = property on="Waveform Chart" class="WFChart (strict)"(error in=w309, "History Data"=waveform(dbl)[][] []) -> (error out=w311:errorcluster)  [unwired: 1 in, 1 out]
          }
          frame "Close" {
            n185 = call <vilib>:"DAQmx Stop Task.vi"("task/channels in"=w316, "error in"=w314) -> ("task out"=w317:refnum<k21>, "error out"=w318:errorcluster)  [unwired: 12 in]
            n186 = Enqueue Element(queue=w315, element="Initialize") -> ()  [unwired: 2 in, 3 out]
            n187 = call <vilib>:"DAQmx Clear Task.vi"("task in"=w317, "error in"=w318) -> ("error out"=w313:errorcluster)  [unwired: 13 in]
          }
          frame "Exit" {
            n188 = call <vilib>:"DAQmx Stop Task.vi"("task/channels in"=w324, "error in"=w320) -> ("task out"=w321:refnum<k21>, "error out"=w322:errorcluster)  [unwired: 12 in]
            n189 = call <vilib>:"DAQmx Clear Task.vi"("task in"=w321, "error in"=w322) -> ("error out"=w323:errorcluster)  [unwired: 13 in]
          }
        }
        "DAQ_IO Error" <- w241
      }
      n190 = while {
        shift-right: [w161] -> _
        shift-left: _ -> [w164]
        shift-right: [w163] -> _
        shift-left: _ -> [w162]
        tunnel: w28 -> [w160]
        stop <- w165 stop-if-true
        n191 = Dequeue Element(queue=w160) -> (queue out=w167:refnum<queue>, element=w166:string)  [unwired: 2 in, 2 out]
        n192 = case shown="\"queryFormat\", Default" w166 {
          tunnel: w167 -> [w177 w186 w195 w205 _ w225 _]
          tunnel: [_ _ _ _ _ _ TRUE] -> w165
          tunnel: [w170 w179 w200 w207 w218 w221 w231] -> w161
          tunnel: w164 -> [_ w189 w193 w208 w219 w223 w229]
          tunnel: [w169 w184 w196 w203 w216 w220 w227] -> w163
          tunnel: w162 -> [_ w188 w197 w204 w217 w224 w228]
          tunnel: "MFC Config" -> [w175 w183 w199 w206 _ _ _]
          frame "Initialize" {
            n193 = Unbundle By Name(w175) -> ("VISA COM Port"=w174:refnum<visa-resource-name>, "baud rate (9600)"=w173:u32)
            n194 = Enqueue Element(queue=w177, element="queryFormat") -> ()  [unwired: 2 in, 3 out]
            n195 = call-poly "VISA Configure Serial Port"("VISA resource name"=w174, "termination char\n(0xA = '\\n' = LF)"=u8 13 ("termination char\n(0xA = '\\n' = LF)"), "Enable Termination\nChar (T)"=TRUE ("Enable Termination\nChar (T)"), "baud rate (9600)"=w173) -> ("VISA resource name out"=w176:refnum<visa-resource-name>, "error out"=w168:errorcluster)  [unwired: 10 in]
            n196 = VISA Clear(VISA resource name=w176, error in (no error)=w168) -> (VISA resource name out=w169:refnum<visa-resource-name>, error out=w170:errorcluster)
          }
          frame "queryFormat", Default {
            n197 = Unbundle By Name(w183) -> ("Device ID's"=w187:string[])
            n198 = Select(t="Close" ("element"), s=w189, f="queryFormat" ("element")) -> (s? t:f=w185:string)
            n199 = Enqueue Element(queue=w186, element=w185) -> ()  [unwired: 2 in, 3 out]
            n200 = call "MFCquery.vi"("error in (no error)"=w189, "Device ID's"=w187, "VISA Refnum in"=w188) -> ("error out"=w180:errorcluster, "Array"=w182:string[], "VISA Refnum out"=w184:refnum<visa-resource-name>)  [unwired: 6 in]
            n201 = call "MFCstringFormat.vi"("error in (no error)"=w180, "Array"=w182) -> ("error out"=w179:errorcluster, "Array out"=→"Array":T12)  [unwired: 7 in]
          }
          frame "tareFlow" {
            n202 = Unbundle By Name(w199) -> ("Device ID's"=w198:string[])
            n203 = Select(t="Close" ("element"), s=w193, f="queryFormat" ("element")) -> (s? t:f=w202:string)
            n204 = Enqueue Element(queue=w195, element=w202) -> ()  [unwired: 2 in, 3 out]
            n205 = call "MFCCMD.vi"("error in (no error)"=w193, "cmd"="v", "Device ID's"=w198, "VISA Refnum in"=w197) -> ("error out"=w200:errorcluster, "VISA Refnum out"=w196:refnum<visa-resource-name>)  [unwired: 6 in]
          }
          frame "tareAbsP" {
            n206 = Unbundle By Name(w206) -> ("Device ID's"=w212:string[])
            n207 = Select(t="Close" ("element"), s=w208, f="queryFormat" ("element")) -> (s? t:f=w213:string)
            n208 = Enqueue Element(queue=w205, element=w213) -> ()  [unwired: 2 in, 3 out]
            n209 = call "MFCCMD.vi"("error in (no error)"=w208, "cmd"="pc", "Device ID's"=w212, "VISA Refnum in"=w204) -> ("error out"=w207:errorcluster, "VISA Refnum out"=w203:refnum<visa-resource-name>)  [unwired: 6 in]
          }
          frame "MFCSet" {
            n210 = local read "MFC Index"() -> (w215:i32)
            n211 = call "MFC_Setpoint.vi"("error in"=w219, "index"=w215, "MFC Set"="MFC Set", "VISA Refnum in"=w217) -> ("error out"=w218:errorcluster, "VISA Refnum out"=w216:refnum<visa-resource-name>)  [unwired: 6 in]
          }
          frame "Close" {
            n212 = VISA Clear(VISA resource name=w224, error in (no error)=w223) -> (VISA resource name out=w220:refnum<visa-resource-name>, error out=w222:errorcluster)
            n213 = VISA Close(VISA resource name=w220, error in (no error)=w222) -> (error out=w221:errorcluster)
            n214 = Enqueue Element(queue=w225, element="Initialize") -> ()  [unwired: 2 in, 3 out]
          }
          frame "Exit" {
            n215 = VISA Clear(VISA resource name=w228, error in (no error)=w229) -> (VISA resource name out=w227:refnum<visa-resource-name>, error out=w230:errorcluster)
            n216 = VISA Close(VISA resource name=w227, error in (no error)=w230) -> (error out=w231:errorcluster)
          }
        }
        "MFC_IO Error" <- w161
        n217 = Wait Until Next ms Multiple(millisecond multiple=u32 100) -> ()  [unwired: 1 out]
      }
      n218 = while {
        tunnel: w17 -> [w53]
        shift-right: [w49] -> _
        shift-left: _ -> [w46]
        shift-right: [w48] -> _
        shift-left: _ -> [w47]
        stop <- w45 stop-if-true
        n219 = Dequeue Element(queue=w53, timeout in ms (-1)=50) -> (queue out=w51:refnum<queue>, element=w52:string)  [unwired: 1 in, 2 out]
        n220 = case shown="\"Timeout\", Default" w52 {
          tunnel: w51 -> [w55 _ w75 _]
          tunnel: [w60 w67 w78 _] -> w49
          tunnel: [w61 w68 w76 _] -> w48
          tunnel: w47 -> [w54 _ _ _]
          tunnel: w46 -> [_ w67 w78 _]
          tunnel: [_ _ _ TRUE] -> w45
          frame "Timeout", Default {
            n221 = Get Date/Time In Seconds() -> (seconds since 1Jan1904=w60:timestamp)
            n222 = Greater?(x=w60, y=w54) -> (0:w59:bool)
            n223 = Select(t="End" ("element"), s=w59, f="Timeout" ("element")) -> (s? t:f=w58:string)
            n224 = Enqueue Element(queue=w55, element=w58) -> ()  [unwired: 2 in, 3 out]
            n225 = property on="Aquire data" class="Bool (strict)"() -> ("Value"=w62:bool)  [unwired: 2 in, 2 out]
            n226 = case shown="False" w62 {
              tunnel: [w63 w66] -> w61
              tunnel: w60 -> [w65 _]
              tunnel: w54 -> [_ w66]
              frame False {
                n227 = To Time Stamp(1:inf) -> (0:w63:timestamp)
                "Start Time" <- w65
              }
              frame True {
              }
            }
          }
          frame "SetEnd" {
            n228 = Multiply(x="Hours to Run", y=1.0) -> (x*y=w69:dbl)
            n229 = Add(x=w69, y=w67) -> (x+y=w68:timestamp)
            "End Time" <- w68
          }
          frame "End" {
            n230 = property on="Timeout Stop" class="Bool (strict)"() -> ("Value"=w73:bool)  [unwired: 2 in, 2 out]
            n231 = To Time Stamp(1:inf) -> (0:w76:timestamp)
            n232 = Not(x=w73) -> (.not. x?=w72:bool)
            n233 = Enqueue Element(queue=w75, element="Timeout") -> ()  [unwired: 2 in, 3 out]
            n234 = property on="Timeout Stop" class="Bool (strict)"("Val(Sgnl)"=w72) -> ()  [unwired: 2 in, 2 out]
          }
          frame "Exit" {
          }
        }
      }
    }
    frame #2 {
      # "In development environment, do not close the panel"
      n235 = property class="App"() -> ("App.Kind"=w528:T9)  [unwired: 2 in, 2 out]
      n236 = Equal?(x=w528, y=T9."Run Time System" ("Application:Kind")) -> (x = y?=w529:bool)
      n237 = case shown="True" w529 {
        frame False {
        }
        frame True {
          n238 = Quit LabVIEW() -> ()  [unwired: 1 in]
        }
      }
    }
  }
